vi "Format PE Name.vi"(1 "String In":string) -> (0 "String Out":string)   [LabVIEW 2020, in "ADAS_IO_Template_MDO.lvclass"]
uses:
  ADAS_IO_Template_MDO.lvclass
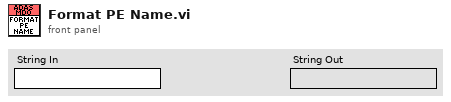
[diagram p1: front panel]
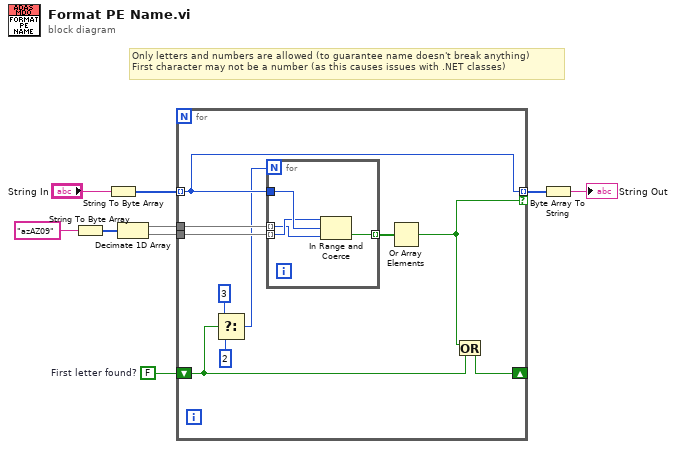
[diagram p0: block diagram]
diagram:
  w1 = FALSE  # First letter found?
  # "Only letters and numbers are allowed (to guarantee name doesn't break anything)\nFirst character may not be a number (as this causes issues with .NET classes)"
  n1 = String To Byte Array(string="azAZ09") -> (unsigned byte array=w8:u8[])
  n2 = String To Byte Array(string="String In") -> (unsigned byte array=w4:u8[])
  n3 = Decimate 1D Array(w8) -> (w7:u8[], w6:u8[])
  n4 = for {
    tunnel: w7 -> [w19]
    tunnel: w6 -> [w18]
    tunnel: w4 -> [w16] mode=indexing
    tunnel: [w16] -> w3 mode=indexing if=w15
    shift-right: [w14] -> _
    shift-left: w1 -> [w13]
    n5 = Select(t=3, s=w13, f=2) -> (s? t:f=w10:i32)
    n6 = for {
      N: w10 -> [_]
      tunnel: w19 -> [w21] mode=indexing
      tunnel: w18 -> [w22] mode=indexing
      tunnel: w16 -> [w23]
      tunnel: [w20] -> w17 mode=indexing
      n7 = In Range and Coerce(upper limit=w22, x=w23, lower limit=w21) -> (In Range?=w20:bool)  [unwired: 1 out]
    }
    n8 = Or Array Elements(Boolean array=w17) -> (logical OR=w15:bool)
    n9 = Or(x=w15, y=w13) -> (x .or. y?=w14:bool)
  }
  n10 = Byte Array To String(unsigned byte array=w3) -> (string=→"String Out":string)
